vi "catch_set_out.vi"(11 "Catch Outputs":T1) -> ()   [LabVIEW 2013]
uses:
  catch_outputs.ctl
  <vilib>/Rock Robotics/WPI/Solenoid/WPI_SolenoidValue.ctl
  <vilib>/Rock Robotics/WPI/Solenoid/WPI_SolenoidSetEnum.vi
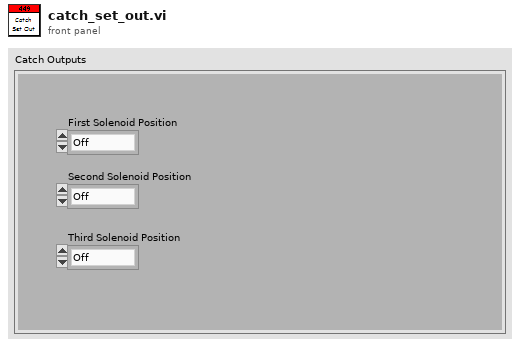
[diagram p1: front panel]
types:
  T1 = typedef "catch_outputs.ctl" = cluster{"First Solenoid Position":T2, "Second Solenoid Position":T2, "Third Solenoid Position":T2}
  T2 = typedef "WPI_SolenoidValue.ctl" = enum16{"Off", "On", "Forward", "Reverse"}
  T3 = typedef "WPI_SolenoidDevRef.ctl" = cluster{"DevStatus":errorcluster, "Solenoid Module":T4, "Forward Solenoid Channel":T5, "Reverse Solenoid Channel":T5}
  T4 = typedef "FPGA_TypedefSolenoidModule.ctl" = enum16{"Solenoid Module 1", "Solenoid Module 2"}
  T5 = typedef "WPI_SolenoidChannel.ctl" = enum8{"Solenoid 1", "Solenoid 2", "Solenoid 3", "Solenoid 4", "Solenoid 5", "Solenoid 6", "Solenoid 7", "Solenoid 8", "Invalid"}
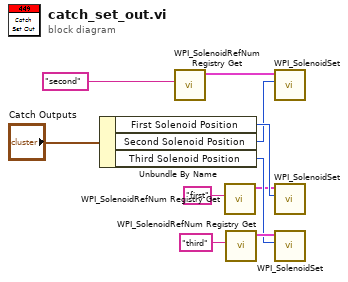
[diagram p0: block diagram]
diagram:
  n1 = Unbundle By Name("Catch Outputs") -> ("First Solenoid Position"=w8:T2, "Second Solenoid Position"=w5:T2, "Third Solenoid Position"=w2:T2)
  n2 = call <vilib>:"WPI_SolenoidRefNum Registry Get.vi"("refnum name"="second") -> ("SolenoidDevRef"=w4:T3)  [unwired: 9 in, 1 out]
  n3 = call <vilib>:"WPI_SolenoidRefNum Registry Get.vi"("refnum name"="first") -> ("SolenoidDevRef"=w1:T3)  [unwired: 9 in, 1 out]
  n4 = call <vilib>:"WPI_SolenoidRefNum Registry Get.vi"("refnum name"="third") -> ("SolenoidDevRef"=w3:T3)  [unwired: 9 in, 1 out]
  n5 = call-poly <vilib>:"WPI_SolenoidSet.vi"("Value"=w5, "SolenoidDevRef"=w4) -> ()  [unwired: 8 in, 2 out]
  n6 = call-poly <vilib>:"WPI_SolenoidSet.vi"("Value"=w8, "SolenoidDevRef"=w1) -> ()  [unwired: 8 in, 2 out]
  n7 = call-poly <vilib>:"WPI_SolenoidSet.vi"("Value"=w2, "SolenoidDevRef"=w3) -> ()  [unwired: 8 in, 2 out]
